vi "Globalvalue1.vi"() -> ()   [LabVIEW 2017]
panel:
  in  "value":i32
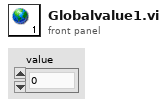
[diagram p1: front panel]
diagram:
